vi "Sequence.CreateStepLoop.vi"(7 "Duration":dbl, 8 "error in (no error)":errorcluster, 9 "Elements":T1[](array[typedef]), 10 "String":string, 11 "String in":string) -> (0 "error out":errorcluster, 3 "Array":refnum<k24>[](array[refnum]))   [LabVIEW 2013, in "Simple Sequence Editor.lvlib"]
uses:
  Simple Sequence Editor.lvlib
  NationalInstruments.VeriStand.RealTimeSequenceDefinitionApi
  Types/Compiled.StepElementProperties.ctl
  Types/ChannelProperties.ctl
  Types/StepTypes.ctl
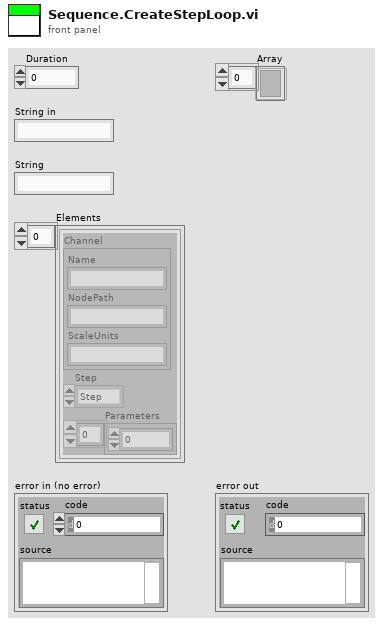
[diagram p1: front panel]
types:
  T1 = typedef "Simple Sequence Editor.lvlib/Compiled.StepElementProperties.ctl" = cluster{"Channel":T2, "Step":T3, "Parameters":dbl[]}
  T2 = typedef "Simple Sequence Editor.lvlib/ChannelProperties.ctl" = cluster{"Name":string, "NodePath":string, "ScaleUnits":string}
  T3 = typedef "Simple Sequence Editor.lvlib/StepTypes.ctl" = enum8{"Step", "iStep", "Ramp", "Unchanged", "Unknown"}
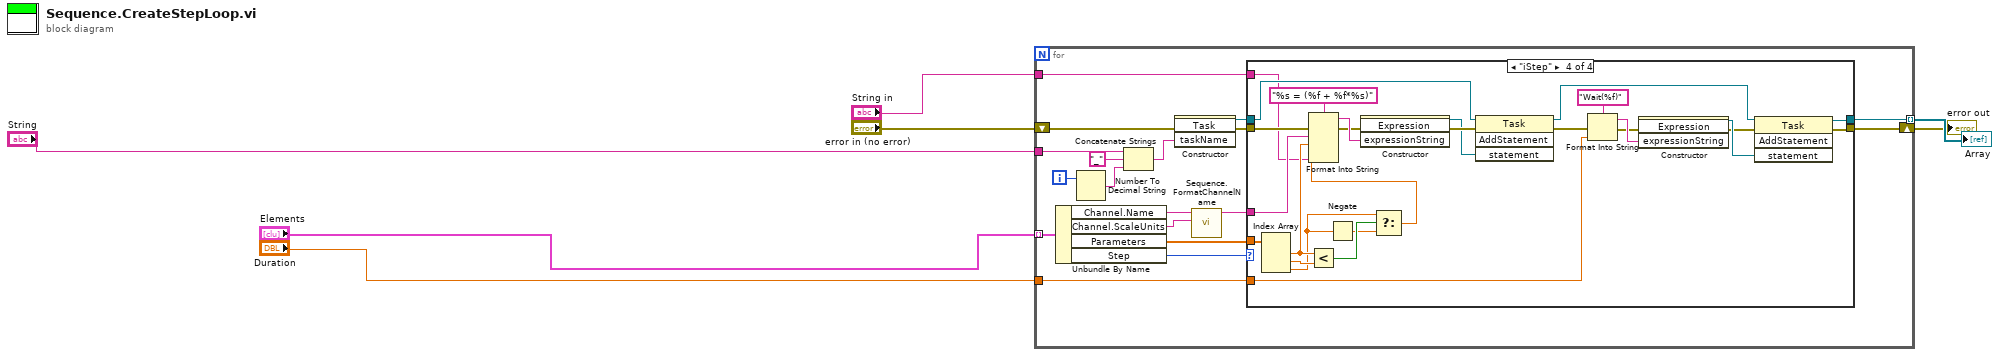
[diagram p0: block diagram]
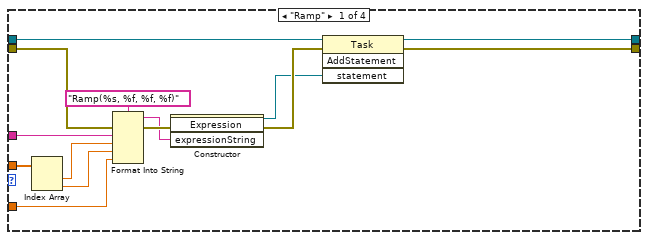
[diagram p2: hidden frame]
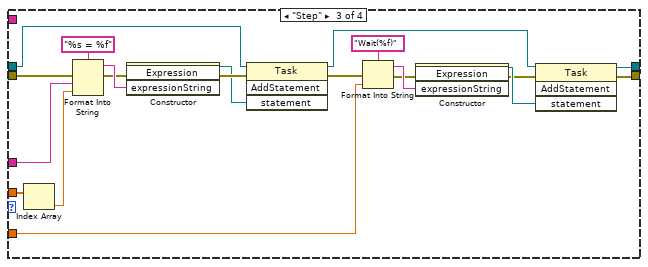
[diagram p4: hidden frame]
diagram:
  n1 = for {
    tunnel: "Elements" -> [w20] mode=indexing
    shift-right: [w11] -> w6
    shift-left: "error in (no error)" -> [w19]
    tunnel: "String" -> [w24]
    tunnel: [w9] -> w7 mode=indexing
    tunnel: "Duration" -> [w15]
    tunnel: "String in" -> [w8]
    i -> [w25]
    n2 = Unbundle By Name(w20) -> ("Channel.Name"=w18:string, "Channel.ScaleUnits"=w17:string, "Parameters"=w14:dbl[], "Step"=w13:T3)
    n3 = Number To Decimal String(number=w25) -> (decimal integer string=w22:string)  [unwired: 1 in]
    n4 = Concatenate Strings(w24, "_" ("string"), w22) -> (w21:string)
    n5 = constructor class="Task"(error in=w19, "taskName"=w21) -> (reference out=w10:refnum<k24>, error out=w12:errorcluster)  [unwired: 2 in, 2 out]
    n6 = call "Sequence.FormatChannelName.vi"("ScaleUnits"=w17, "Name"=w18) -> ("String"=w16:string)  [unwired: 9 in]
    n7 = case shown="\"iStep\"" w13 {
      tunnel: w16 -> [w38 _ w60 w86]
      tunnel: w14 -> [w37 _ w59 w85]
      tunnel: w15 -> [w34 _ w50 w77]
      tunnel: [w28 w40 w44 w71] -> w11
      tunnel: w12 -> [w33 w40 w57 w84]
      tunnel: w10 -> [w30 w41 w49 w76]
      tunnel: [w27 w41 w42 w69] -> w9
      tunnel: w8 -> [_ _ _ w62]
      frame "Ramp" {
        n8 = Index Array(array=w37) -> (element #1=w36:dbl, element #2=w35:dbl)  [unwired: 2 in]
        n9 = Format Into String(format string="Ramp(%s, %f, %f, %f)" ("expressionString"), error in=w33, w38, w36, w35, w34) -> (resulting string=w26:string, error out=w29:errorcluster)  [unwired: 1 in]
        n10 = constructor class="Expression"(error in=w29, "expressionString"=w26) -> (reference out=w31:refnum<k24>, error out=w32:errorcluster)  [unwired: 2 in, 2 out]
        n11 = invoke class="Task" method="AddStatement"(reference=w30, error in=w32, "statement"=w31) -> (reference out=w27:refnum<k24>, error out=w28:errorcluster)  [unwired: 1 in, 2 out]
      }
      frame "Unchanged", Default {
      }
      frame "Step" {
        n12 = Index Array(array=w59) -> (element=w58:dbl)  [unwired: 1 in]
        n13 = Format Into String(format string="%s = %f" ("expressionString"), error in=w57, w60, w58) -> (resulting string=w54:string, error out=w45:errorcluster)  [unwired: 1 in]
        n14 = constructor class="Expression"(error in=w45, "expressionString"=w54) -> (reference out=w55:refnum<k24>, error out=w56:errorcluster)  [unwired: 2 in, 2 out]
        n15 = invoke class="Task" method="AddStatement"(reference=w49, error in=w56, "statement"=w55) -> (reference out=w43:refnum<k24>, error out=w46:errorcluster)  [unwired: 1 in, 2 out]
        n16 = Format Into String(format string="Wait(%f)", error in=w46, w50) -> (resulting string=w48:string, error out=w47:errorcluster)  [unwired: 1 in]
        n17 = constructor class="Expression"(error in=w47, "expressionString"=w48) -> (reference out=w53:refnum<k24>, error out=w52:errorcluster)  [unwired: 2 in, 2 out]
        n18 = invoke class="Task" method="AddStatement"(reference=w43, error in=w52, "statement"=w53) -> (reference out=w42:refnum<k24>, error out=w44:errorcluster)  [unwired: 1 in, 2 out]
      }
      frame "iStep" {
        n19 = Index Array(array=w85) -> (element #1=w68:dbl, element #2=w67:dbl, element #3=w64:dbl)  [unwired: 3 in]
        n20 = Less?(x=w68, y=w67) -> (x < y?=w66:bool)
        n21 = Negate(x=w64) -> (-x=w65:dbl)
        n22 = Select(t=w64, s=w66, f=w65) -> (s? t:f=w63:dbl)
        n23 = Format Into String(format string="%s = (%f + %f*%s)" ("expressionString"), error in=w84, w86, w68, w63, w62) -> (resulting string=w81:string, error out=w72:errorcluster)  [unwired: 1 in]
        n24 = constructor class="Expression"(error in=w72, "expressionString"=w81) -> (reference out=w82:refnum<k24>, error out=w83:errorcluster)  [unwired: 2 in, 2 out]
        n25 = invoke class="Task" method="AddStatement"(reference=w76, error in=w83, "statement"=w82) -> (reference out=w70:refnum<k24>, error out=w73:errorcluster)  [unwired: 1 in, 2 out]
        n26 = Format Into String(format string="Wait(%f)", error in=w73, w77) -> (resulting string=w75:string, error out=w74:errorcluster)  [unwired: 1 in]
        n27 = constructor class="Expression"(error in=w74, "expressionString"=w75) -> (reference out=w80:refnum<k24>, error out=w79:errorcluster)  [unwired: 2 in, 2 out]
        n28 = invoke class="Task" method="AddStatement"(reference=w70, error in=w79, "statement"=w80) -> (reference out=w69:refnum<k24>, error out=w71:errorcluster)  [unwired: 1 in, 2 out]
      }
    }
  }
  "Array" <- w7
  "error out" <- w6
